vi "SET DRIVE FRAME.vi"(10 "drive frame":T1) -> ()   [LabVIEW 2023]
uses:
  ctrl defs/ctrl DRIVING FRAME selector.ctl
  Global odometry.vi
  <vilib>/Rock Robotics/Network Tables/NT Write String.vi
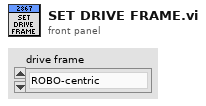
[diagram p1: front panel]
types:
  T1 = typedef "ctrl DRIVING FRAME selector.ctl" = enum16{"ROBO-centric", "FLD-centric"}
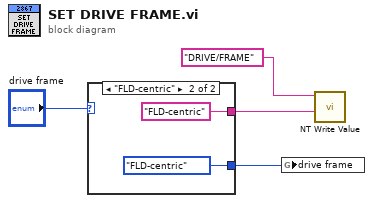
[diagram p0: block diagram]
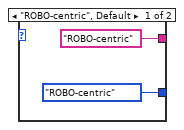
[diagram p2: hidden frame]
diagram:
  n1 = case shown="\"FLD-centric\"" "drive frame" {
    tunnel: ["ROBO-centric" ("value") "FLD-centric" ("value")] -> w2
    tunnel: [ctrl_DRIVING_FRAME_selector."ROBO-centric" ("drive frame") ctrl_DRIVING_FRAME_selector."FLD-centric" ("drive frame")] -> w1
    frame "ROBO-centric", Default {
    }
    frame "FLD-centric" {
    }
  }
  n2 = global write "Global odometry.vi" "drive frame"(w1) -> ()
  n3 = call-poly <vilib>:"NT Write Value.vi"("value"=w2, "name"="DRIVE/FRAME") -> ()  [unwired: 9 in, 1 out]
